vi "secondary field controller.vi"() -> ()   [LabVIEW 2010]
uses:
  <vilib>/DAQmx/write.llb/DAQmx Write (Analog Wfm 1Chan NSamp).vi
  <vilib>/Utility/file.llb/Write To Spreadsheet File (string).vi
  <vilib>/DAQmx/create/channels.llb/DAQmx Create Channel (AO-Voltage-Basic).vi
  <vilib>/DAQmx/configure/timing.llb/DAQmx Timing (Use Waveform).vi
  <vilib>/daqmx/miscellaneous.llb/DAQmx Fill In Error Info.vi
  <vilib>/gmath/NI_Gmath.lvlib
panel:
  in  "name":string
  in  "saved":i32(listbox)
  in  "delete":bool
  in  "save":bool
  in  "load":bool
  in  "sweeps":u32=1
  in  "functions":T1(array[cluster])=[{"f(x)"="x", "min x"=-1.0, "max x"=1.0, "steps"=500.0}]
  in  "period (s)":dbl=1.0 step=1.0 format="%#_3f"
  in  "record periodically":bool
  in  "record single sweeps":bool
  in  "log file":path
  in  "finite":bool
  in  "range (V pk-to-pk)":dbl=2.0 step=1.0 format="%#_3f"
  out "modulation":waveform(dbl)(graph)
  in  "DAC channel":tag="Dev4/ao0"
  in  "run":bool
  in  "R&S address":string="29"
  in  "steps / second":u32=10000 step=1
  in  "amplitude (mV)":i32=275
  in  "modulation (kHz)":i32=400 step=1
  in  "center frequency (MHz)":dbl=213.0 min=0.0 step=0.001 format="%#_6f"
  # "RF settings"
  # "sweep settings"
  # "FINITE"
  # "ON"
  # "CONTINUOUS"
  # "full modulation range\nis [-1, 1] V\n\npi = 3.14159\n2*pi = 6.28319"
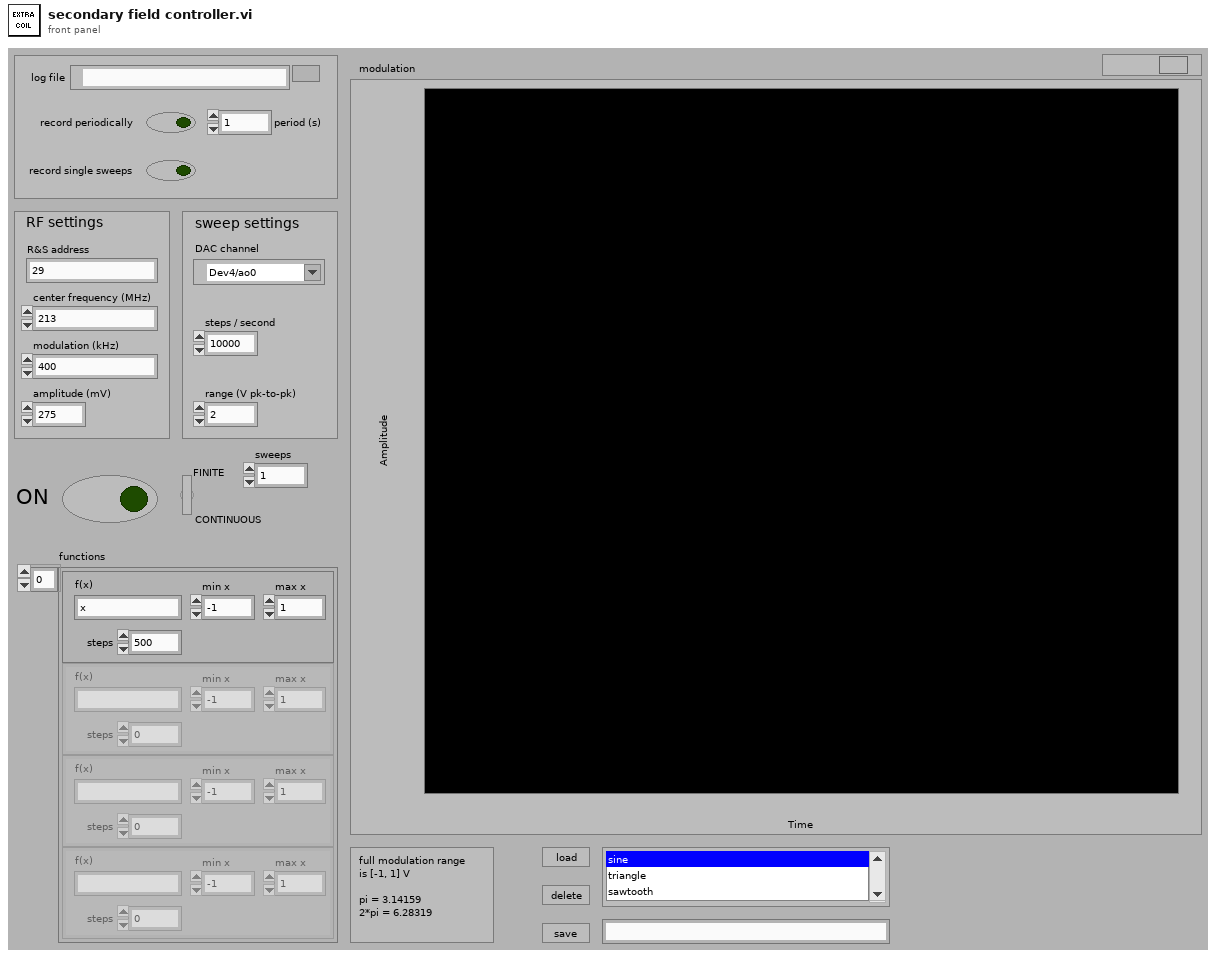
[diagram p1: front panel]
types:
  T1 = cluster{"f(x)":string, "min x":dbl, "max x":dbl, "steps":dbl}[]
  T2 = enum16{"initialize", "idle", "update sweep settings", "run", "stop"}
  T3 = cluster{"f(x)":string, "min x":dbl, "max x":dbl, "steps":dbl}[][]
  T4 = cluster{string[], cluster{"f(x)":string, "min x":dbl, "max x":dbl, "steps":dbl}[][]}
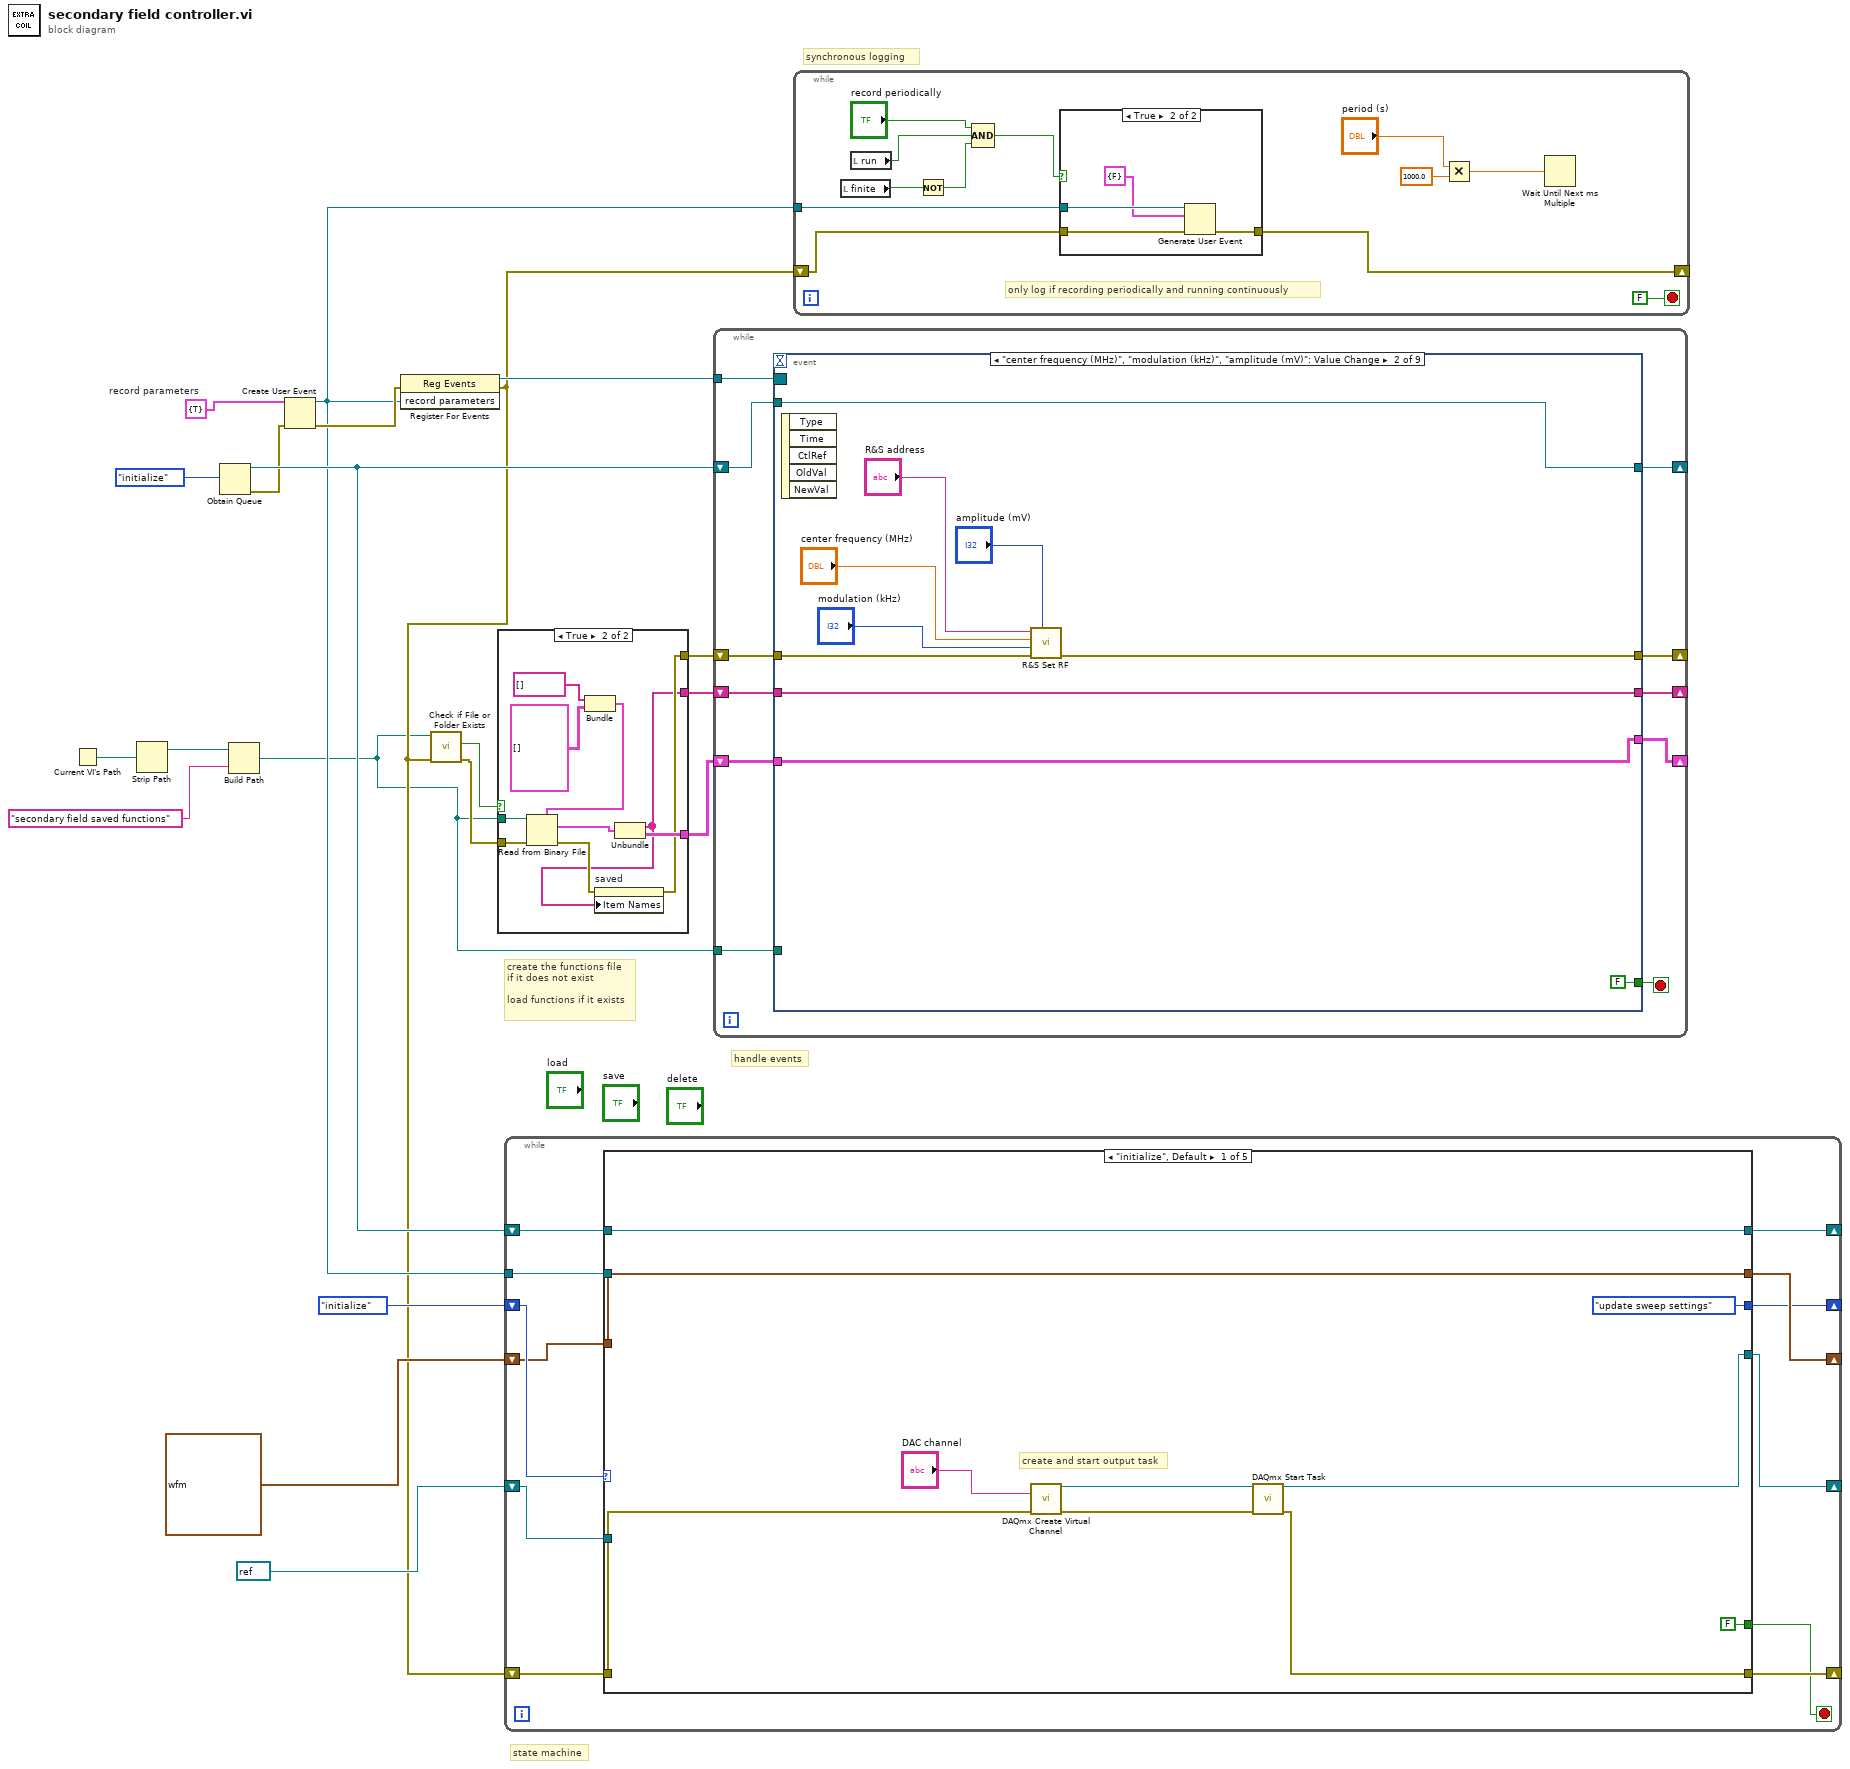
[diagram p0: block diagram]
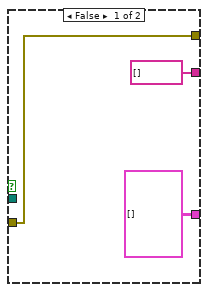
[diagram p2: hidden frame]
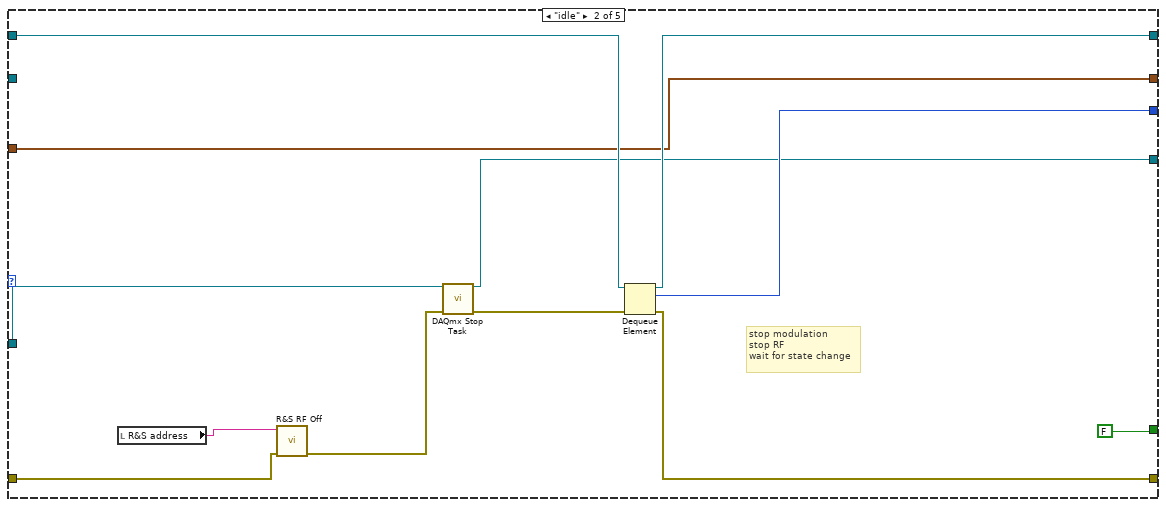
[diagram p4: hidden frame]
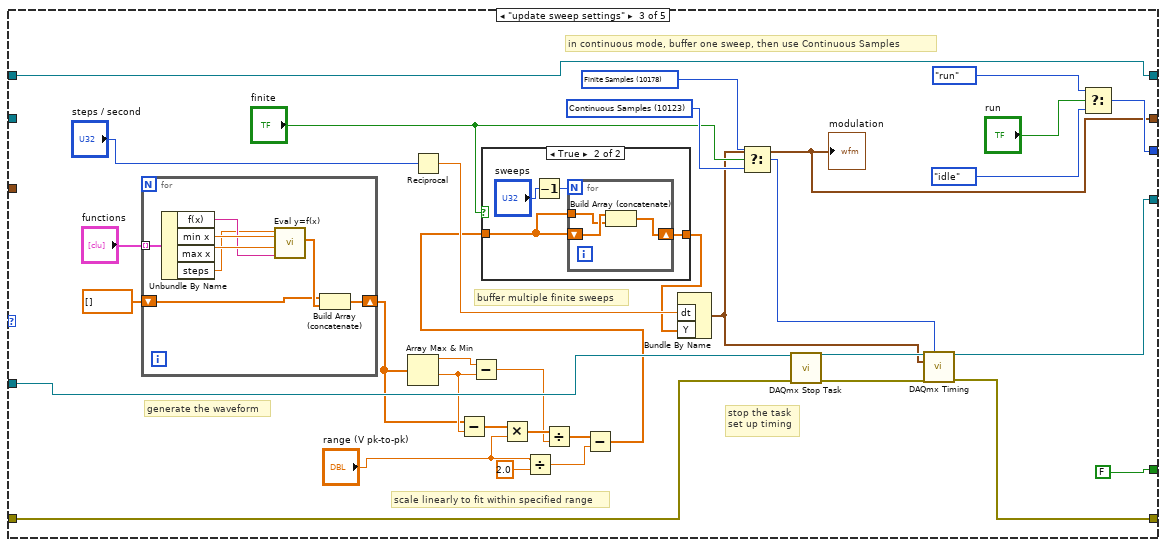
[diagram p5: hidden frame]
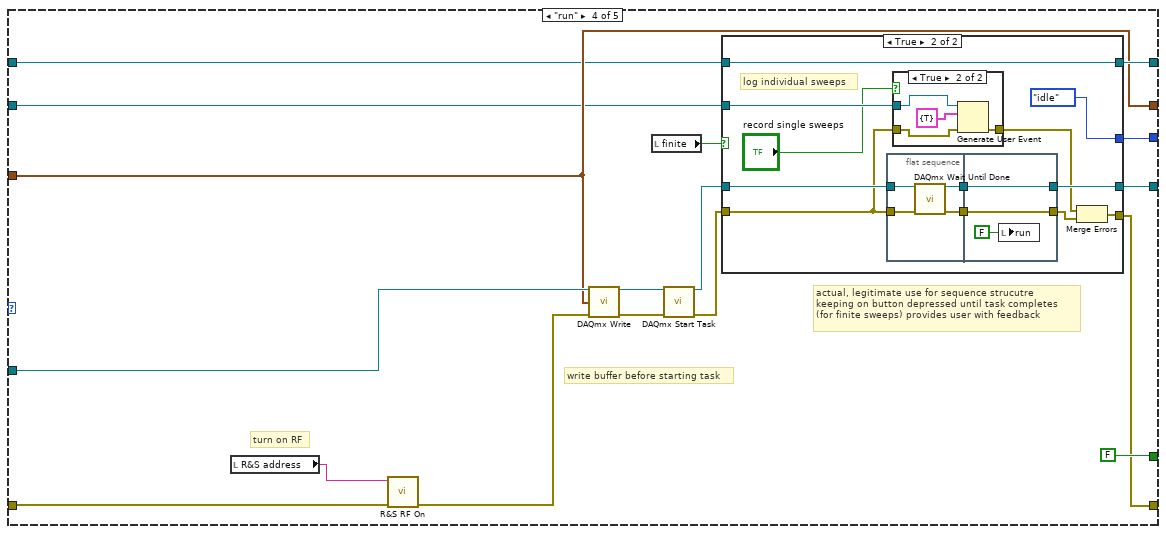
[diagram p7: hidden frame]
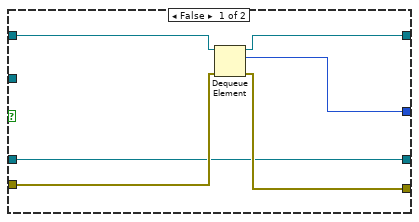
[diagram p8: hidden frame]
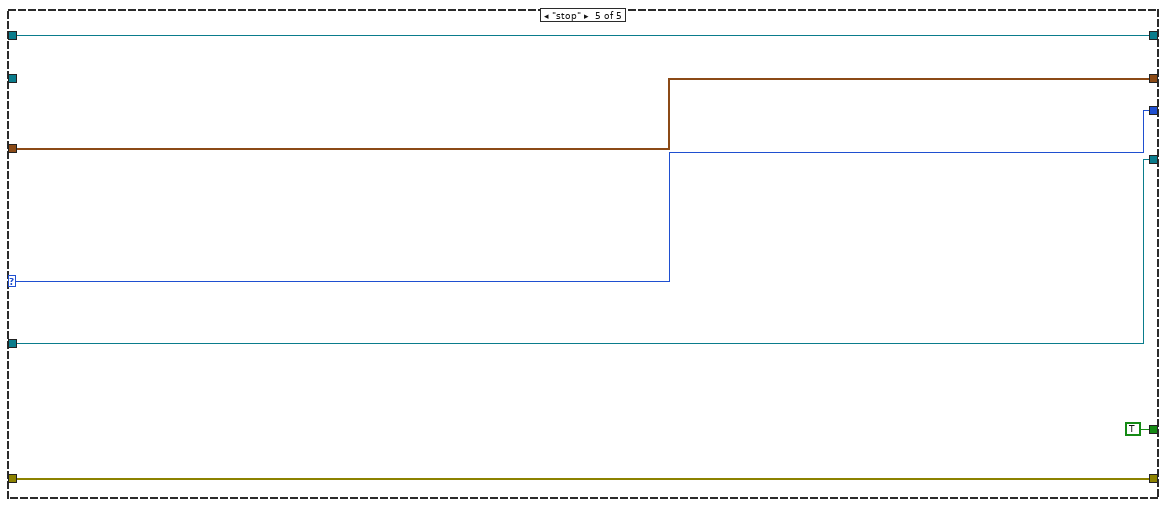
[diagram p10: hidden frame]
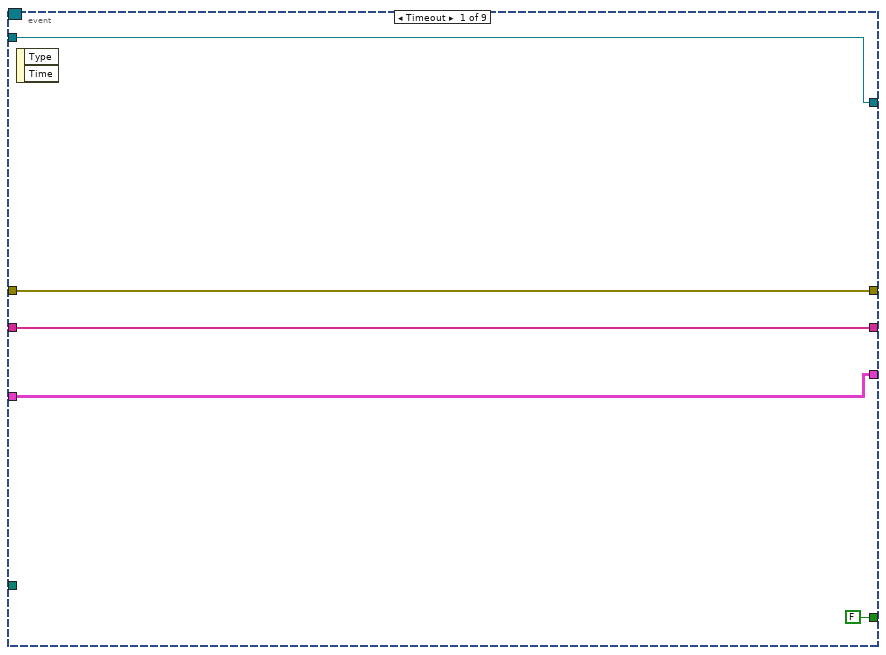
[diagram p11: hidden frame]
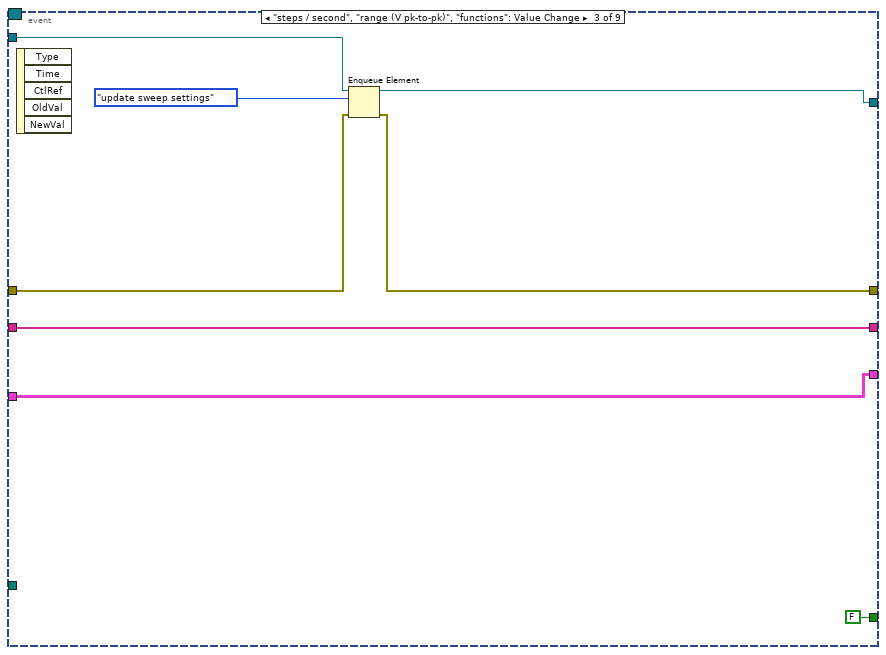
[diagram p12: hidden frame]
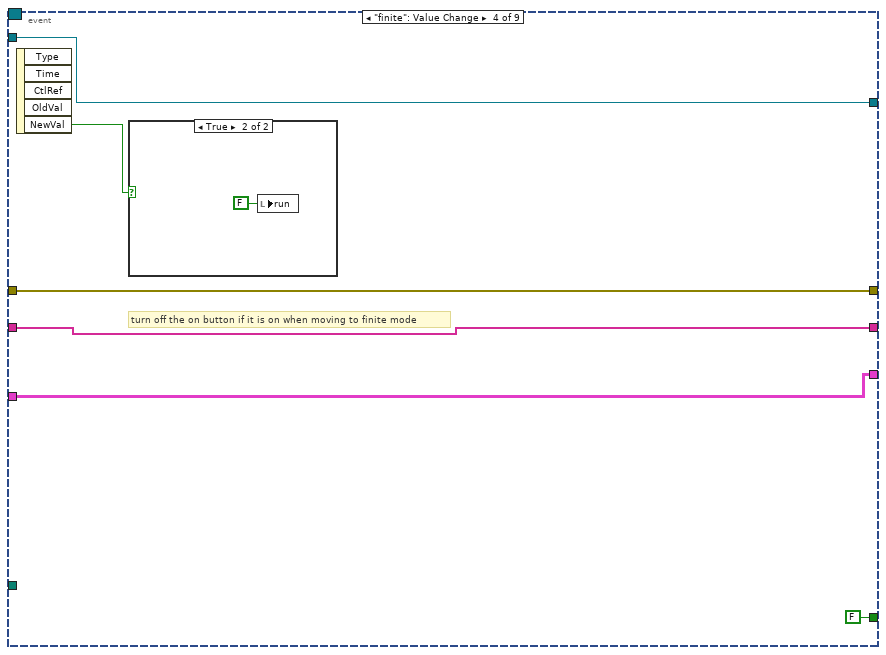
[diagram p13: hidden frame]
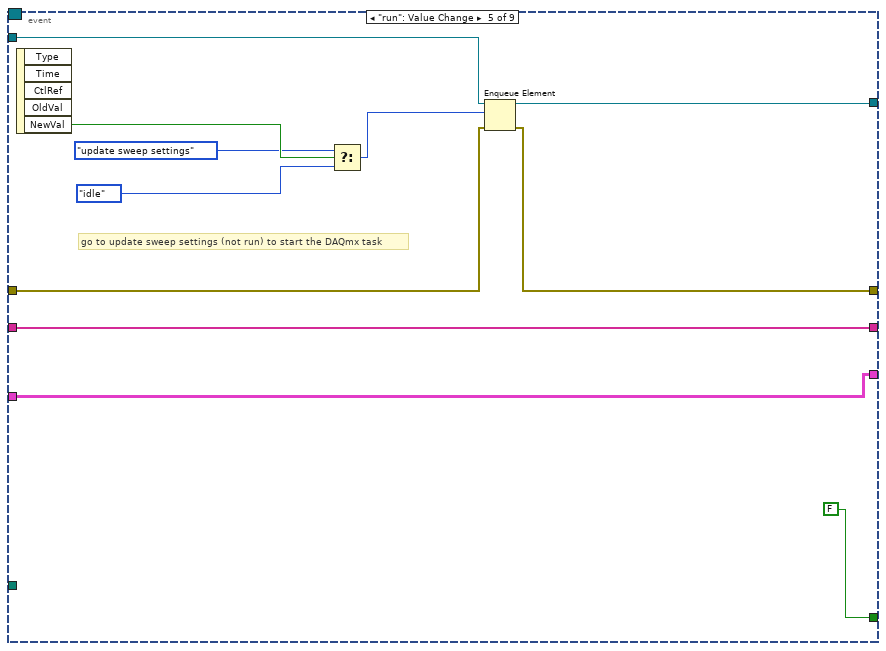
[diagram p15: hidden frame]
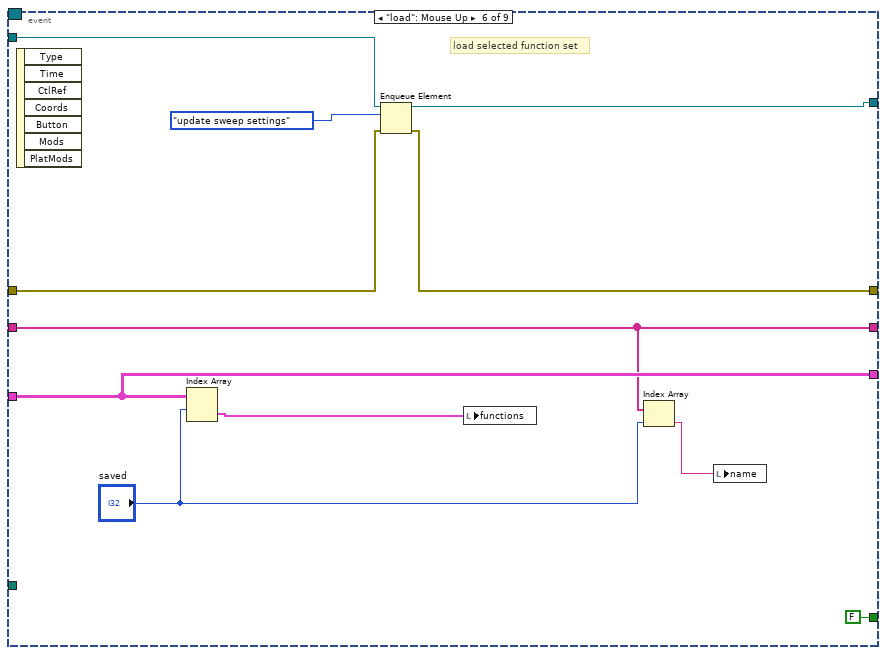
[diagram p16: hidden frame]
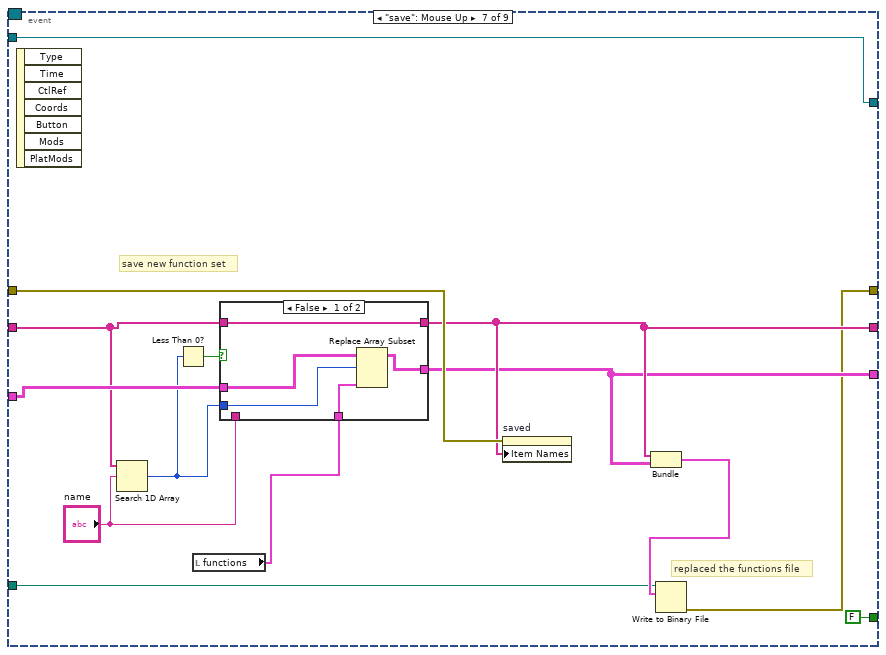
[diagram p17: hidden frame]
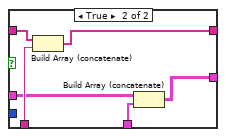
[diagram p18: hidden frame]
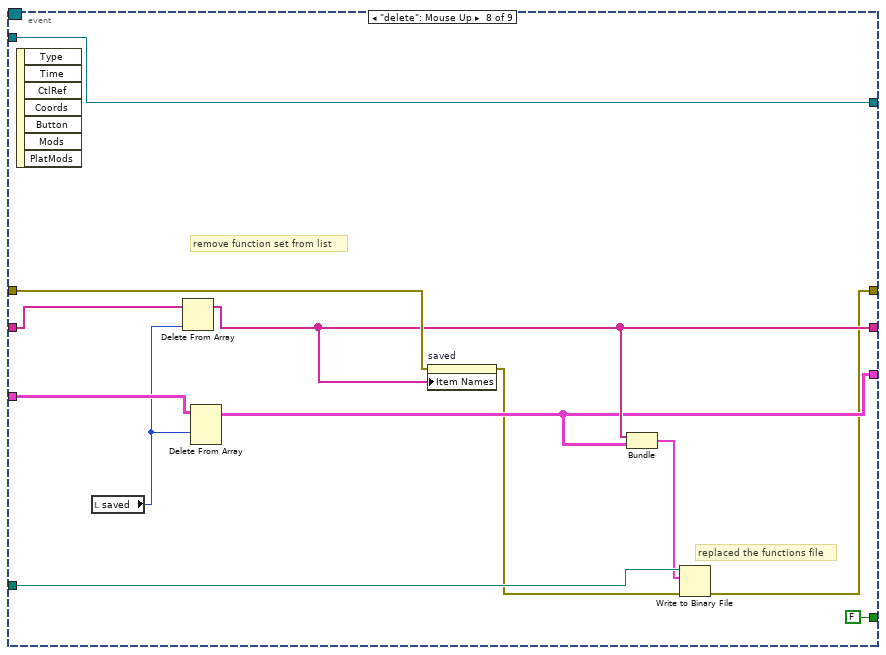
[diagram p19: hidden frame]
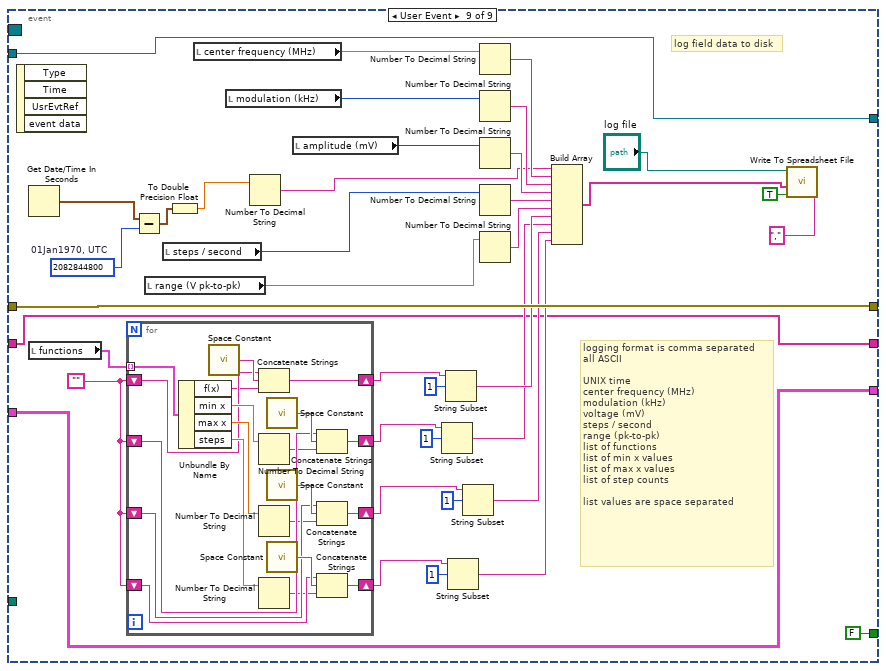
[diagram p20: hidden frame]
diagram:
  w12 = cluster{"event data":bool} {"event data"=TRUE}  # record parameters
  # "state machine"
  # "handle events"
  # "create the functions file\nif it does not exist\n\nload functions if it exists"
  # "synchronous logging"
  n1 = Current VI's Path() -> (path=w4:path)
  n2 = Strip Path(path=w4) -> (stripped path=w3:path)  [unwired: 1 out]
  n3 = Obtain Queue(element data type=T2."initialize") -> (queue out=w19:refnum<queue>, error out=w13:errorcluster)  [unwired: 4 in, 1 out]
  n4 = Build Path(base path=w3, name or relative path="secondary field saved functions") -> (appended path=w1:path)
  n5 = Create User Event(user event datatype=w12, error in=w13) -> (user event=w11:refnum<user-event>, error out=w14:errorcluster)
  n6 = register-events(error in=w14, w11) -> (reference out=w15:refnum<event-registration>, error out=w10:errorcluster)  [unwired: 1 in]
  n7 = call <vilib>:"Check if File or Folder Exists.vi"("error in (no error)"=w10, "path"=w1) -> ("error out"=w8:errorcluster, "file or folder exists?"=w9:bool)  [unwired: 7 in, 1 out]
  n8 = case shown="True" w9 {
    tunnel: w8 -> [w21 w30]
    tunnel: [string[] [] w24] -> w7
    tunnel: [T3 [] w28] -> w6
    tunnel: [w21 w25] -> w5
    tunnel: w1 -> [_ w27]
    frame False {
    }
    frame True {
      n9 = Bundle(string[] [], T3 []) -> (w31:T4)  [unwired: 1 in]
      n10 = Read from Binary File(5:w31, 8:w30, 11:w27) -> (0:w26:errorcluster, 2:w29:T4)  [unwired: 3 in, 2 out]
      n11 = Unbundle(w29) -> (w24:string[], w28:T3)
      n12 = property on="saved" class="LstBox (strict)"(error in=w26, "Item Names"=w24) -> (error out=w25:errorcluster)  [unwired: 1 in, 1 out]
    }
  }
  n13 = while {
    shift-right: [w40] -> _
    shift-left: w19 -> [w41]
    shift-right: [w43] -> _
    shift-left: w10 -> [w44]
    shift-right: [w39] -> _
    shift-left: T2."initialize" -> [w45]
    shift-right: [w42] -> _
    shift-left: waveform(dbl) {"t0"=timestamp(0 s since 1904-01-01), "dt"=1.0, "Y"=[]} ("signal out") -> [w38]
    shift-right: [w35] -> _
    shift-left: refnum<k21> refnum ("task out") -> [w37]
    tunnel: w11 -> [w34]
    stop <- w36 stop-if-true
    n14 = case shown="\"initialize\", Default" w45 {
      selector: w45 -> [_ _ _ _ w166]
      tunnel: w44 -> [w53 w58 w89 w119 w169]
      tunnel: [w52 w65 w92 w121 w169] -> w43
      tunnel: [w51 w63 w68 w125 w168] -> w42
      tunnel: w41 -> [w49 w67 w96 w124 w167]
      tunnel: [w49 w66 w96 w129 w167] -> w40
      tunnel: [T2."update sweep settings" w64 w97 w123 w166] -> w39
      tunnel: w38 -> [w51 w63 _ w125 w168]
      tunnel: w37 -> [_ w60 w88 w133 w164]
      tunnel: [FALSE FALSE FALSE FALSE TRUE] -> w36
      tunnel: [w46 w59 w75 w122 w164] -> w35
      tunnel: w34 -> [_ _ _ w120 _]
      frame "initialize", Default {
        # "create and start output task"
        n15 = call-poly <vilib>:"DAQmx Create Virtual Channel.vi"("physical channels"="DAC channel", "error in"=w53) -> ("task out"=w48:refnum<k21>, "error out"=w47:errorcluster)  [unwired: 12 in]
        n16 = call <vilib>:"DAQmx Start Task.vi"("task/channels in"=w48, "error in"=w47) -> ("task out"=w46:refnum<k21>, "error out"=w52:errorcluster)  [unwired: 12 in]
      }
      frame "idle" {
        # "stop modulation\nstop RF\nwait for state change"
        n17 = local read "R&S address"() -> (w56:string)
        n18 = call "R&S RF Off.vi"("error in (no error)"=w58, "address"=w56) -> ("error out"=w57:errorcluster)  [unwired: 4 in, 1 out]
        n19 = call <vilib>:"DAQmx Stop Task.vi"("task/channels in"=w60, "error in"=w57) -> ("task out"=w59:refnum<k21>, "error out"=w61:errorcluster)  [unwired: 12 in]
        n20 = Dequeue Element(queue=w67, error in (no error)=w61) -> (queue out=w66:refnum<queue>, element=w64:T2, error out=w65:errorcluster)  [unwired: 1 in, 1 out]
      }
      frame "update sweep settings" {
        w77 = 10123 items=["Finite Samples"=10178, "Continuous Samples"=10123, "Hardware Timed Single Point"=12522] ("sample mode")
        w78 = 10178 items=["Finite Samples"=10178, "Continuous Samples"=10123, "Hardware Timed Single Point"=12522] ("sample mode")
        # "stop the task\nset up timing"
        # "in continuous mode, buffer one sweep, then use Continuous Samples"
        # "buffer multiple finite sweeps"
        # "scale linearly to fit within specified range"
        # "generate the waveform"
        n21 = for {
          tunnel: "functions" -> [w116] mode=indexing
          shift-right: [w110] -> w72
          shift-left: dbl[] [] -> [w109]
          n22 = Unbundle By Name(w116) -> ("f(x)"=w113:string, "min x"=w115:dbl, "max x"=w114:dbl, "steps"=w112:dbl)
          n23 = call <vilib>:"Eval y=f(x).vi"("formula"=w113, "end"=w114, "start"=w115, "number of points"=w112) -> ("Y Values"=w111:dbl[])  [unwired: 3 out]
          n24 = Build Array (concatenate)(w109, w111) -> (w110:dbl[])
        }
        n25 = Array Max & Min(array=w72) -> (max value=w86:dbl, min value=w85:dbl)  [unwired: 2 out]
        n26 = Reciprocal(x="steps / second") -> (1/x=w90:dbl)
        n27 = Subtract(x=w72, y=w85) -> (x-y=w87:dbl[])
        n28 = Subtract(x=w86, y=w85) -> (x-y=w83:dbl)
        n29 = Multiply(x=w87, y="range (V pk-to-pk)") -> (x*y=w84:dbl[])
        n30 = Divide(x="range (V pk-to-pk)", y=2.0) -> (x/y=w80:dbl)
        n31 = Divide(x=w84, y=w83) -> (x/y=w82:dbl[])
        n32 = Subtract(x=w82, y=w80) -> (x-y=w70:dbl[])
        n33 = case shown="True" "finite" {
          tunnel: w70 -> [w101 w104]
          tunnel: [w101 w102] -> w69
          frame False {
          }
          frame True {
            n34 = Decrement(x="sweeps") -> (x-1=w103:u32)
            n35 = for {
              N: w103 -> [_]
              shift-right: [w106] -> w102
              shift-left: w104 -> [w108]
              tunnel: w104 -> [w107]
              n36 = Build Array (concatenate)(w108, w107) -> (w106:dbl[])
            }
          }
        }
        n37 = Bundle By Name("dt"=w90, "Y"=w69) -> (w68:waveform(dbl))  [unwired: 1 in]
        "modulation" <- w68
        n38 = Select(t=w78, s="finite", f=w77) -> (s? t:f=w76:i32)
        n39 = call <vilib>:"DAQmx Stop Task.vi"("task/channels in"=w88, "error in"=w89) -> ("task out"=w93:refnum<k21>, "error out"=w94:errorcluster)  [unwired: 12 in]
        n40 = call-poly <vilib>:"DAQmx Timing.vi"("task/channels in"=w93, "sample mode"=w76, "waveform"=w68, "error in"=w94) -> ("task out"=w75:refnum<k21>, "error out"=w92:errorcluster)  [unwired: 10 in]
        n41 = Select(t=T2."run" ("element"), s="run", f=T2."idle" ("element")) -> (s? t:f=w97:T2)
      }
      frame "run" {
        # "turn on RF"
        # "write buffer before starting task"
        # "actual, legitimate use for sequence strucutre\nkeeping on button depressed until task completes\n(for finite sweeps) provides user with feedback"
        n42 = local read "R&S address"() -> (w117:string)
        n43 = call "R&S RF On.vi"("error in (no error)"=w119, "address"=w117) -> ("error out"=w118:errorcluster)  [unwired: 4 in, 1 out]
        n44 = call-poly <vilib>:"DAQmx Write.vi"("task/channels in"=w133, "data"=w125, "error in"=w118) -> ("task out"=w131:refnum<k21>, "error out"=w130:errorcluster)  [unwired: 10 in, 1 out]
        n45 = local read "finite"() -> (w126:bool)
        n46 = call <vilib>:"DAQmx Start Task.vi"("task/channels in"=w131, "error in"=w130) -> ("task out"=w128:refnum<k21>, "error out"=w127:errorcluster)  [unwired: 12 in]
        n47 = case shown="True" w126 {
          tunnel: [w136 w143] -> w121
          tunnel: [w138 w150] -> w129
          tunnel: w128 -> [w134 w151]
          tunnel: w127 -> [w137 w144]
          tunnel: w124 -> [w139 w150]
          tunnel: [w135 T2."idle" ("element")] -> w123
          tunnel: [w134 w148] -> w122
          tunnel: w120 -> [_ w145]
          frame False {
            n48 = Dequeue Element(queue=w139, error in (no error)=w137) -> (queue out=w138:refnum<queue>, element=w135:T2, error out=w136:errorcluster)  [unwired: 1 in, 1 out]
          }
          frame True {
            # "log individual sweeps"
            n49 = flat-sequence {
              tunnel: w151 -> [w160]
              tunnel: w144 -> [w159]
              tunnel: [w158] -> w147
              tunnel: [w157] -> w146
              tunnel: [w162] -> w148
              tunnel: [w163] -> w142
              tunnel: w147 -> [w163]
              tunnel: w146 -> [w162]
              frame #0 {
                n50 = call <vilib>:"DAQmx Wait Until Done.vi"("task/channels in"=w160, "error in"=w159) -> ("task out"=w157:refnum<k21>, "error out"=w158:errorcluster)  [unwired: 12 in]
              }
              frame #1 {
                n51 = local write "run"(FALSE ("run")) -> ()
              }
            }
            n52 = case shown="True" "record single sweeps" {
              tunnel: w145 -> [_ w153]
              tunnel: w144 -> [w152 w154]
              tunnel: [w152 w156] -> w141
              frame False {
              }
              frame True {
                n53 = Generate User Event(user event=w153, event data cluster=cluster{"event data":bool} {"event data"=TRUE} ("event data"), error in=w154) -> (error out=w156:errorcluster)  [unwired: 1 out]
              }
            }
            n54 = Merge Errors(w141, w142) -> (w143:errorcluster)
          }
        }
      }
      frame "stop" {
      }
    }
  }
  n55 = while {
    shift-right: [w177] -> _
    shift-left: w19 -> [w180]
    shift-right: [w178] -> _
    shift-left: w5 -> [w179]
    tunnel: w15 -> [w175]
    shift-right: [w171] -> _
    shift-left: w6 -> [w174]
    shift-right: [w172] -> _
    shift-left: w7 -> [w173]
    tunnel: w1 -> [w170]
    stop <- w176 stop-if-true
    n56 = event shown="[1] \"center frequency (MHz)\", \"modulation (kHz)\", \"amplitude (mV)\": Value Change" {
      selector: w175 -> [_ _ _ _ _ _ _ _ _]
      dyn-events: _ -> [_ _ _ _ _ _ _ _ _]
      timeout: _ -> [_ _ _ _ _ _ _ _ _]
      tunnel: w180 -> [w185 w190 w203 w209 w221 w231 w244 w265 w293]
      tunnel: w179 -> [w184 w195 w201 w208 w220 w230 w242 w266 w295]
      tunnel: [w184 w186 w200 w208 w219 w229 w238 w258 w295] -> w178
      tunnel: [w185 w190 w199 w209 w218 w228 w244 w265 w293] -> w177
      tunnel: [FALSE FALSE FALSE FALSE FALSE FALSE FALSE FALSE FALSE] -> w176
      tunnel: w174 -> [w181 w187 w196 w204 w211 w226 w246 w269 w270]
      tunnel: w173 -> [w182 w188 w197 w205 w212 w224 w236 w268 w271]
      tunnel: [w182 w188 w197 w205 w212 w224 w241 w263 w271] -> w172
      tunnel: [w181 w187 w196 w204 w211 w226 w240 w262 w270] -> w171
      tunnel: w170 -> [_ _ _ _ _ _ w237 w261 _]
      event Timeout {
        n57 = event-data() -> ()  [unwired: 1 in, 2 out]
      }
      event "center frequency (MHz)", "modulation (kHz)", "amplitude (mV)": Value Change {
        n58 = event-data() -> ()  [unwired: 1 in, 5 out]
        n59 = call "R&S Set RF.vi"("amplitude (mV)"="amplitude (mV)", "error in (no error)"=w195, "modulation (kHz)"="modulation (kHz)", "center frequency (MHz)"="center frequency (MHz)", "address"="R&S address") -> ("error out"=w186:errorcluster)  [unwired: 2 in, 1 out]
      }
      event "steps / second", "range (V pk-to-pk)", "functions": Value Change {
        n60 = event-data() -> ()  [unwired: 1 in, 5 out]
        n61 = Enqueue Element(queue=w203, element=T2."update sweep settings", error in (no error)=w201) -> (queue out=w199:refnum<queue>, error out=w200:errorcluster)  [unwired: 1 in, 1 out]
      }
      event "finite": Value Change {
        # "turn off the on button if it is on when moving to finite mode"
        n62 = event-data() -> ("NewVal"=w207:bool)  [unwired: 1 in, 4 out]
        n63 = case shown="True" w207 {
          frame False {
          }
          frame True {
            n64 = local write "run"(FALSE ("run")) -> ()
          }
        }
      }
      event "run": Value Change {
        # "go to update sweep settings (not run) to start the DAQmx task"
        n65 = event-data() -> ("NewVal"=w216:bool)  [unwired: 1 in, 4 out]
        n66 = Select(t=T2."update sweep settings", s=w216, f=T2."idle") -> (s? t:f=w217:T2)
        n67 = Enqueue Element(queue=w221, element=w217, error in (no error)=w220) -> (queue out=w218:refnum<queue>, error out=w219:errorcluster)  [unwired: 1 in, 1 out]
      }
      event "load": Mouse Up {
        # "load selected function set"
        n68 = event-data() -> ()  [unwired: 1 in, 7 out]
        n69 = Index Array(array=w226, index (row)="saved") -> (element=w232:T1)  [unwired: 1 in]
        n70 = Enqueue Element(queue=w231, element=T2."update sweep settings", error in (no error)=w230) -> (queue out=w228:refnum<queue>, error out=w229:errorcluster)  [unwired: 1 in, 1 out]
        n71 = local write "functions"(w232) -> ()
        n72 = Index Array(array=w224, index="saved") -> (element=w222:string)
        n73 = local write "name"(w222) -> ()
      }
      event "save": Mouse Up {
        # "save new function set"
        # "replaced the functions file"
        n74 = event-data() -> ()  [unwired: 1 in, 7 out]
        n75 = Search 1D Array(1D array=w236, element="name") -> (index of element=w233:i32)  [unwired: 1 in]
        n76 = Less Than 0?(x=w233) -> (x < 0?=w234:bool)
        n77 = local read "functions"() -> (w245:T1)
        n78 = case shown="False" w234 {
          tunnel: w236 -> [w247 w257]
          tunnel: "name" -> [_ w256]
          tunnel: w246 -> [w251 w255]
          tunnel: w245 -> [w249 w254]
          tunnel: [w247 w253] -> w241
          tunnel: [w248 w252] -> w240
          tunnel: w233 -> [w250 _]
          frame False {
            n79 = Replace Array Subset(array=w251, new element=w249, index (row)=w250) -> (w248:T3)  [unwired: 1 in]
          }
          frame True {
            n80 = Build Array (concatenate)(w257, w256) -> (w253:string[])
            n81 = Build Array (concatenate)(w255, w254) -> (w252:T3)
          }
        }
        n82 = property on="saved" class="LstBox (strict)"(error in=w242, "Item Names"=w241) -> ()  [unwired: 1 in, 2 out]
        n83 = Bundle(w241, w240) -> (w239:T4)  [unwired: 1 in]
        n84 = Write to Binary File(file (use dialog)=w237, data=w239) -> (error out=w238:errorcluster)  [unwired: 4 in, 2 out]
      }
      event "delete": Mouse Up {
        # "replaced the functions file"
        # "remove function set from list"
        n85 = event-data() -> ()  [unwired: 1 in, 7 out]
        n86 = local read "saved"() -> (w267:i32)
        n87 = Delete From Array(array=w268, index=w267) -> (array with subset deleted=w263:string[])  [unwired: 1 in, 1 out]
        n88 = Delete From Array(array=w269, index (row)=w267) -> (array with subset deleted=w262:T3)  [unwired: 2 in, 1 out]
        n89 = property on="saved" class="LstBox (strict)"(error in=w266, "Item Names"=w263) -> (error out=w259:errorcluster)  [unwired: 1 in, 1 out]
        n90 = Bundle(w263, w262) -> (w260:T4)  [unwired: 1 in]
        n91 = Write to Binary File(file (use dialog)=w261, data=w260, error in=w259) -> (error out=w258:errorcluster)  [unwired: 3 in, 2 out]
      }
      event User Event {
        w284 = ""
        w292 = u64 2082844800  # 01Jan1970, UTC
        # "log field data to disk"
        # "logging format is comma separated\nall ASCII\n\nUNIX time\ncenter frequency (MHz)\nmodulation (kHz)\nvoltage (mV)\nsteps / second\nrange (pk-to-pk)\nlist of functions\nlist of min x values\nlist of max x values\nlist of step counts\n\nlist values are space separated"
        n92 = event-data() -> ()  [unwired: 1 in, 4 out]
        n93 = Get Date/Time In Seconds() -> (seconds since 1Jan1904=w291:timestamp)
        n94 = local read "functions"() -> (w285:T1)
        n95 = for {
          tunnel: w285 -> [w327] mode=indexing
          shift-right: [w322] -> w279
          shift-left: w284 -> [w315]
          shift-right: [w321] -> w278
          shift-left: w284 -> [w314]
          shift-right: [w320] -> w277
          shift-left: w284 -> [w313]
          shift-right: [w319] -> w276
          shift-left: w284 -> [w312]
          n96 = Unbundle By Name(w327) -> ("f(x)"=w311:string, "min x"=w318:dbl, "max x"=w317:dbl, "steps"=w316:dbl)
          n97 = call <vilib>:"Space Constant.vi"() -> ("String"=w326:string)
          n98 = Concatenate Strings(w315, w326, w311) -> (w322:string)
          n99 = Number To Decimal String(number=w318) -> (decimal integer string=w310:string)  [unwired: 1 in]
          n100 = Number To Decimal String(number=w317) -> (decimal integer string=w309:string)  [unwired: 1 in]
          n101 = Number To Decimal String(number=w316) -> (decimal integer string=w308:string)  [unwired: 1 in]
          n102 = call <vilib>:"Space Constant.vi"() -> ("String"=w325:string)
          n103 = call <vilib>:"Space Constant.vi"() -> ("String"=w324:string)
          n104 = call <vilib>:"Space Constant.vi"() -> ("String"=w323:string)
          n105 = Concatenate Strings(w314, w325, w310) -> (w321:string)
          n106 = Concatenate Strings(w313, w324, w309) -> (w320:string)
          n107 = Concatenate Strings(w312, w323, w308) -> (w319:string)
        }
        n108 = Subtract(x=w291, y=w292) -> (x-y=w290:timestamp)
        n109 = local read "range (V pk-to-pk)"() -> (w286:dbl)
        n110 = local read "steps / second"() -> (w287:u32)
        n111 = To Double Precision Float(number=w290) -> (double precision float=w289:dbl)
        n112 = local read "center frequency (MHz)"() -> (w305:dbl)
        n113 = local read "modulation (kHz)"() -> (w304:i32)
        n114 = Number To Decimal String(number=w289) -> (decimal integer string=w288:string)  [unwired: 1 in]
        n115 = local read "amplitude (mV)"() -> (w303:i32)
        n116 = String Subset(string=w278, offset (0)=1) -> (substring=w272:string)  [unwired: 1 in]
        n117 = String Subset(string=w279, offset (0)=1) -> (substring=w275:string)  [unwired: 1 in]
        n118 = String Subset(string=w276, offset (0)=1) -> (substring=w273:string)  [unwired: 1 in]
        n119 = String Subset(string=w277, offset (0)=1) -> (substring=w274:string)  [unwired: 1 in]
        n120 = Number To Decimal String(number=w305) -> (decimal integer string=w302:string)  [unwired: 1 in]
        n121 = Number To Decimal String(number=w304) -> (decimal integer string=w301:string)  [unwired: 1 in]
        n122 = Number To Decimal String(number=w303) -> (decimal integer string=w300:string)  [unwired: 1 in]
        n123 = Number To Decimal String(number=w287) -> (decimal integer string=w299:string)  [unwired: 1 in]
        n124 = Number To Decimal String(number=w286) -> (decimal integer string=w298:string)  [unwired: 1 in]
        n125 = Build Array(w288, w302, w301, w300, w299, w298, w275, w272, w274, w273) -> (w297:string[])
        n126 = call-poly <vilib>:"Write To Spreadsheet File.vi"("delimiter (\\t)"="," ("delimiter (\\t)"), "append to file? (new file:F)"=TRUE, "1D data"=w297, "file path (dialog if empty)"="log file") -> ()  [unwired: 4 in, 1 out]
      }
    }
  }
  n127 = while {
    shift-right: [w337] -> _
    shift-left: w10 -> [w339]
    tunnel: w11 -> [w338]
    stop <- FALSE stop-if-true
    # "only log if recording periodically and running continuously"
    n128 = local read "finite"() -> (w330:bool)
    n129 = local read "run"() -> (w331:bool)
    n130 = Not(x=w330) -> (.not. x?=w329:bool)
    n131 = Compound Arithmetic op=AND("record periodically", w331, w329) -> (w328:bool)
    n132 = case shown="True" w328 {
      tunnel: w339 -> [w340 w344]
      tunnel: w338 -> [_ w343]
      tunnel: [w340 w341] -> w337
      frame False {
      }
      frame True {
        n133 = Generate User Event(user event=w343, event data cluster=cluster{"event data":bool} {"event data"=FALSE} ("event data"), error in=w344) -> (error out=w341:errorcluster)  [unwired: 1 out]
      }
    }
    n134 = Multiply(x="period (s)", y=1000.0) -> (x*y=w333:dbl)
    n135 = Wait Until Next ms Multiple(millisecond multiple=w333) -> ()  [unwired: 1 out]
  }
